vi "Modify Custom Waveform.vi"(11 "Custom Wfm Config":T1={"File Path"="", "Sample Rate (Hz)"=10000000.0, "Read From"=0, "Pre Delay (s)"=0.0, "Post Delay (s)"=0.0, "Scale"=1.0} {"Scale" min=0.0 format="%#_6p"}) -> (2 "Waveform Modified?":bool, 3 "Modified Waveform":waveform(dbl))   [LabVIEW 2025, in "TDMS Waveform Creator UI.lvlib"]
uses:
  TDMS Waveform Creator UI.lvlib
panel:
  out "File Path":path
  in  "Scale":dbl=1.0 min=0.0 format="%#_6p"
  in  "Post Delay (s)":dbl min=0.0 format="%#_6p"
  in  "Pre Delay (s)":dbl min=0.0 format="%#_6p"
  in  "File Type":enum32{"CSV", "TDMS", "TDM"}(radio)
  in  "Read From":i32 caption="Read From Row/Wfm Index" min=0
  in  "Load File":bool
  in  "Suggest Naming?":bool=TRUE
  in  "Waveform Name":string
  in  "Cancel":bool
  in  "OK":bool
  out "Actual Sample Size":i32
  out "Actual Duration (s)":dbl format="%#_6p"
  out "Waveform Preview":waveform(dbl)(graph)
  in  "Sample Rate (Hz)":dbl=10000000.0 min=0.0 format="%#_6p"
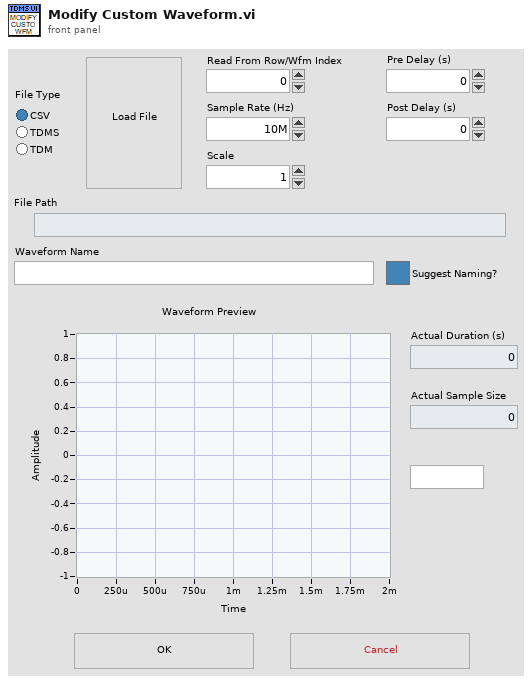
[diagram p1: front panel]
types:
  T1 = cluster{"File Path":string, "Sample Rate (Hz)":dbl, "Read From":i32, "Pre Delay (s)":dbl, "Post Delay (s)":dbl, "Scale":dbl}
  T2 = cluster{"pattern (all files)":string, "pattern label":string, "prompt":string}
  T3 = cluster{"pattern (all files)":string, "pattern label":string, "prompt":string}[]
  T4 = enum8{"Enabled", "Disabled", "Disabled and Grayed Out"}
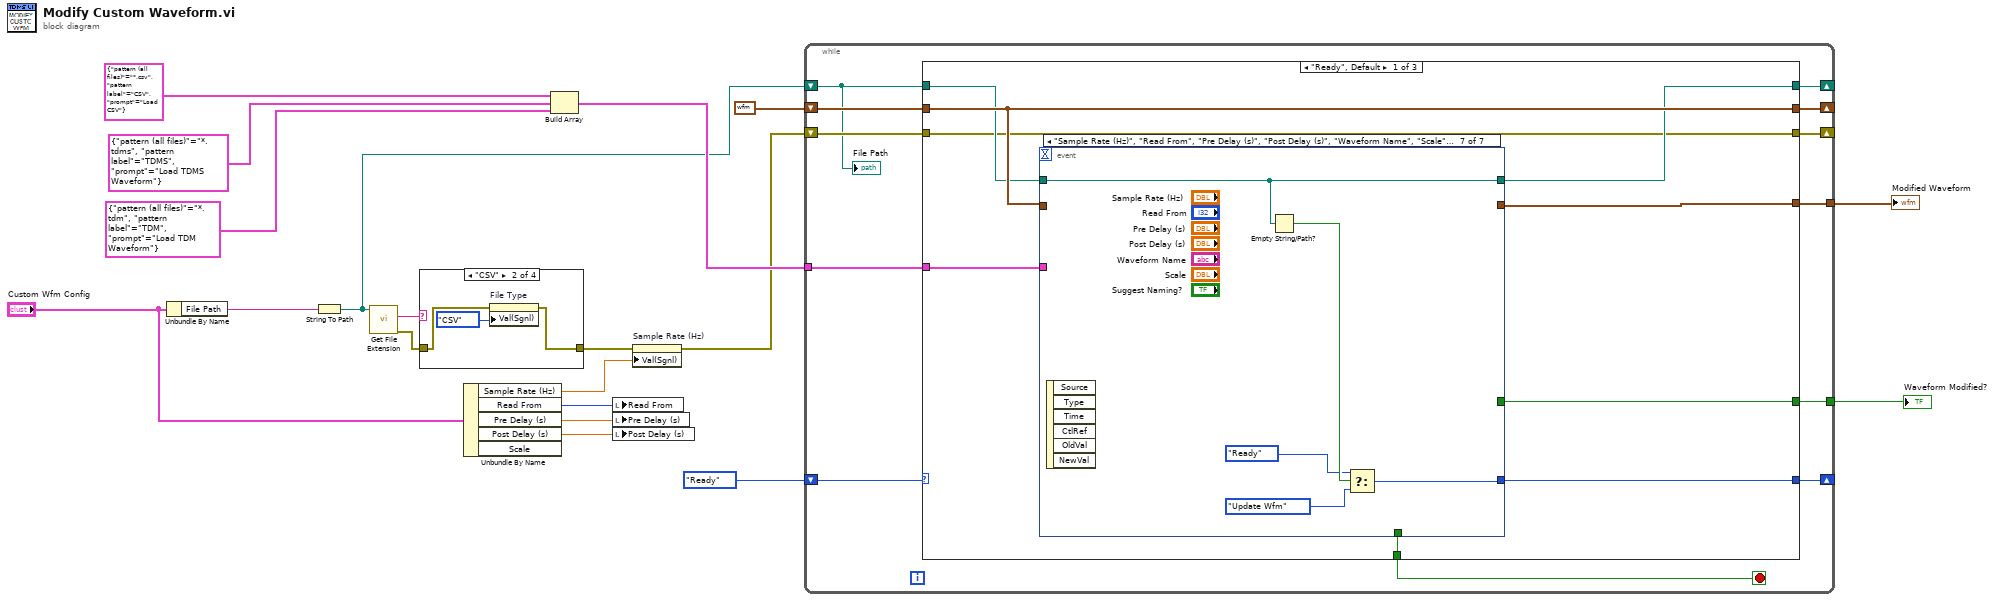
[diagram p0: block diagram]
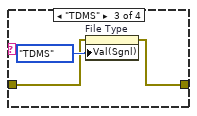
[diagram p3: hidden frame]
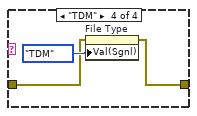
[diagram p4: hidden frame]
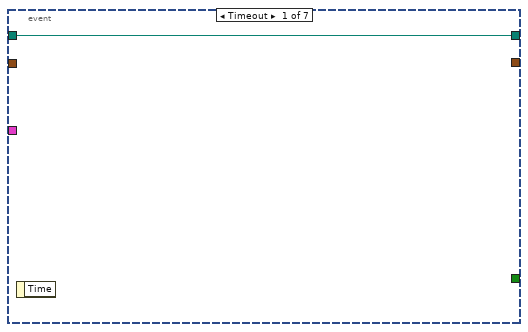
[diagram p5: hidden frame]
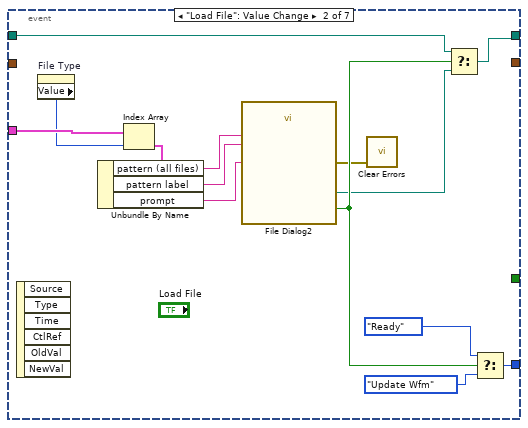
[diagram p6: hidden frame]
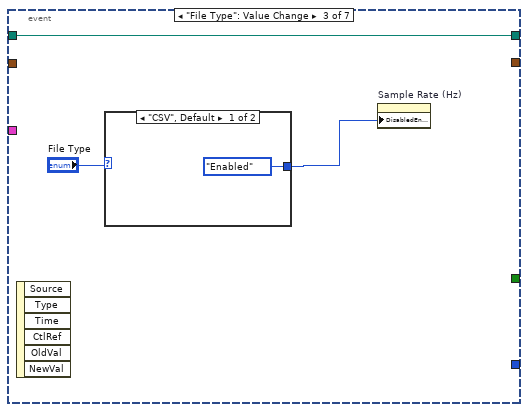
[diagram p7: hidden frame]
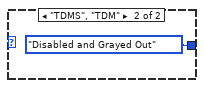
[diagram p8: hidden frame]
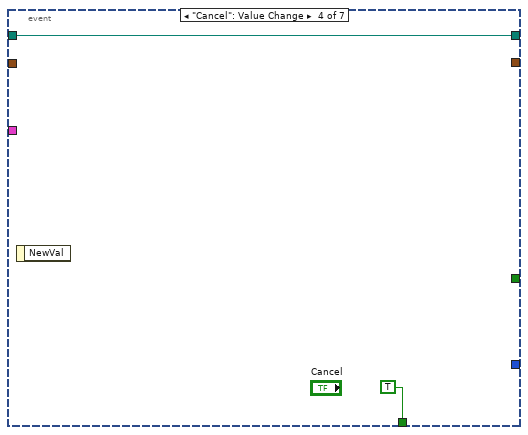
[diagram p9: hidden frame]
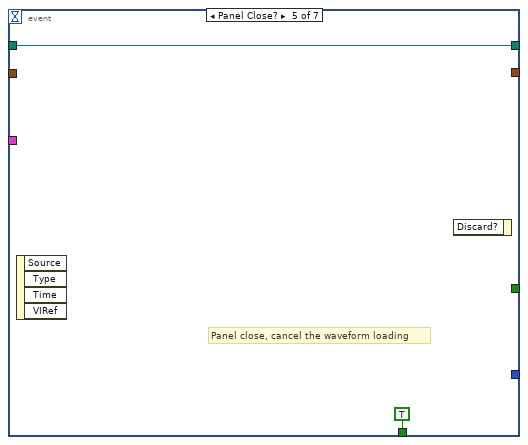
[diagram p10: hidden frame]
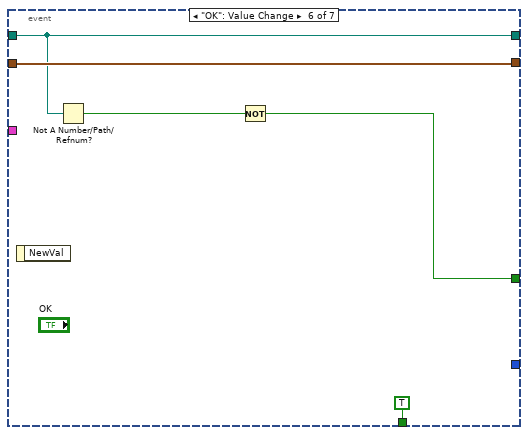
[diagram p11: hidden frame]
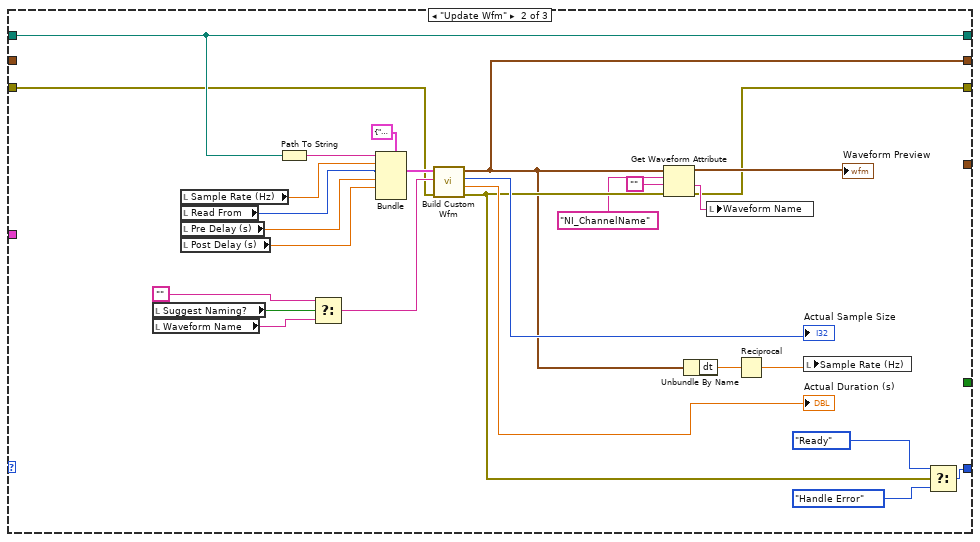
[diagram p12: hidden frame]
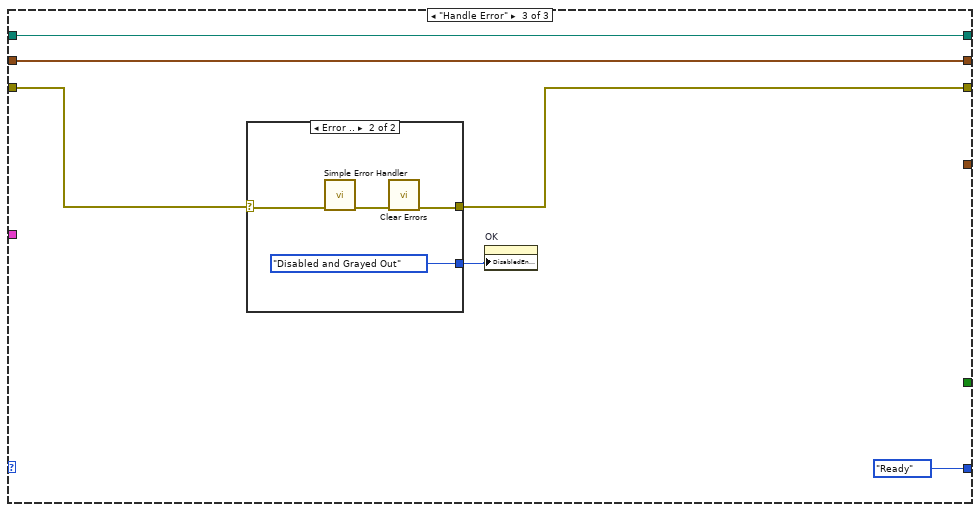
[diagram p13: hidden frame]
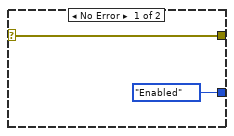
[diagram p14: hidden frame]
diagram:
  n1 = Unbundle By Name("Custom Wfm Config") -> ("File Path"=w11:string)
  n2 = String To Path(string=w11) -> (path=w10:path)
  n3 = call <vilib>:"Get File Extension.vi"("file"=w10) -> ("error out"=w8:errorcluster, "lowercase file extension"=w9:string)  [unwired: 6 in, 3 out]
  n4 = case shown="\"CSV\"" w9 {
    tunnel: w8 -> [w20 w21 w24 w27]
    tunnel: [w20 w22 w25 w28] -> w7
    frame Default {
    }
    frame "CSV" {
      n5 = property on="File Type" class="RadioBtnsControl (strict)"(error in=w21, "Val(Sgnl)"=enum32{"CSV", "TDMS", "TDM"}."CSV" ("Value (Signaling)")) -> (error out=w22:errorcluster)  [unwired: 1 in, 1 out]
    }
    frame "TDMS" {
      n6 = property on="File Type" class="RadioBtnsControl (strict)"(error in=w24, "Val(Sgnl)"=enum32{"CSV", "TDMS", "TDM"}."TDMS" ("Value (Signaling)")) -> (error out=w25:errorcluster)  [unwired: 1 in, 1 out]
    }
    frame "TDM" {
      n7 = property on="File Type" class="RadioBtnsControl (strict)"(error in=w27, "Val(Sgnl)"=enum32{"CSV", "TDMS", "TDM"}."TDM" ("Value (Signaling)")) -> (error out=w28:errorcluster)  [unwired: 1 in, 1 out]
    }
  }
  n8 = Unbundle By Name("Custom Wfm Config") -> ("Sample Rate (Hz)"=w4:dbl, "Read From"=w3:i32, "Pre Delay (s)"=w2:dbl, "Post Delay (s)"=w1:dbl)  [unwired: 1 out]
  n9 = Build Array(T2 {"pattern (all files)"="*.csv", "pattern label"="CSV", "prompt"="Load CSV"}, T2 {"pattern (all files)"="*.tdms", "pattern label"="TDMS", "prompt"="Load TDMS Waveform"}, T2 {"pattern (all files)"="*.tdm", "pattern label"="TDM", "prompt"="Load TDM Waveform"}) -> (w13:T3)
  n10 = local write "Read From"(w3) -> ()
  n11 = local write "Pre Delay (s)"(w2) -> ()
  n12 = local write "Post Delay (s)"(w1) -> ()
  n13 = property on="Sample Rate (Hz)" class="DigNum (strict)"(error in=w7, "Val(Sgnl)"=w4) -> (error out=w6:errorcluster)  [unwired: 1 in, 1 out]
  n14 = while {
    tunnel: [w40] -> w19
    shift-right: [w38] -> _
    shift-left: enum16{"Ready", "Update Wfm", "Handle Error"}."Ready" -> [w39]
    shift-right: [w37] -> _
    shift-left: w10 -> [w30]
    shift-right: [w35] -> _
    shift-left: waveform(dbl) {"t0"=timestamp(0 s since 1904-01-01), "dt"=1.0, "Y"=[]} ("Output Waveform") -> [w36]
    tunnel: [w34] -> w16
    tunnel: w13 -> [w33]
    shift-right: [w31] -> _
    shift-left: w6 -> [w32]
    stop <- w41 stop-if-true
    n15 = case shown="\"Ready\", Default" w39 {
      tunnel: [w50 _ _] -> w41
      tunnel: [w49 _ _] -> w40
      tunnel: [w48 w111 enum16{"Ready", "Update Wfm", "Handle Error"}."Ready"] -> w38
      tunnel: w30 -> [w45 w108 w116]
      tunnel: [w44 w108 w116] -> w37
      tunnel: w36 -> [w47 _ w117]
      tunnel: [w47 w88 w117] -> w35
      tunnel: [w46 _ _] -> w34
      tunnel: w33 -> [w43 _ _]
      tunnel: w32 -> [w42 w91 w114]
      tunnel: [w42 w92 w113] -> w31
      frame "Ready", Default {
        n16 = event shown="[6] \"Sample Rate (Hz)\", \"Read From\", \"Pre Delay (s)\", \"Post Delay (s)\", \"Waveform Name\", \"Scale\", \"Suggest Naming?\": Value Change" {
          selector: _ -> [_ _ _ _ _ _ _]
          dyn-events: _ -> [_ _ _ _ _ _ _]
          timeout: _ -> [_ _ _ _ _ _ _]
          tunnel: [_ _ _ TRUE TRUE TRUE _] -> w50
          tunnel: [_ _ _ _ _ w75 _] -> w49
          tunnel: [_ w65 _ _ _ _ w84] -> w48
          tunnel: w47 -> [_ _ _ _ _ w78 _]
          tunnel: [_ _ _ _ _ w78 _] -> w46
          tunnel: w45 -> [w51 w63 w68 w71 w74 w77 w83]
          tunnel: [w51 w61 w68 w71 w74 w77 w83] -> w44
          tunnel: w43 -> [_ w60 _ _ _ _ _]
          event Timeout {
            n17 = event-data() -> ()  [unwired: 1 in, 1 out]
          }
          event "Load File": Value Change {
            n18 = event-data() -> ()  [unwired: 1 in, 6 out]
            n19 = property on="File Type" class="RadioBtnsControl (strict)"() -> ("Value"=w55:enum32{"CSV", "TDMS", "TDM"})  [unwired: 2 in, 2 out]
            n20 = Index Array(array=w60, index=w55) -> (element=w59:T2)
            n21 = Unbundle By Name(w59) -> ("pattern (all files)"=w58:string, "pattern label"=w57:string, "prompt"=w56:string)
            n22 = call "File Dialog2"("prompt"=w56, "pattern (all files)"=w58, "pattern label"=w57) -> ("selected path"=w62:path, "cancelled"=w64:bool, "error out"=w54:errorcluster)  [unwired: 9 in, 1 out]
            n23 = call <vilib>:"Clear Errors.vi"("error in (no error)"=w54) -> ()  [unwired: 5 in, 2 out]
            n24 = Select(t=w63, s=w64, f=w62) -> (s? t:f=w61:path)
            n25 = Select(t=enum16{"Ready", "Update Wfm", "Handle Error"}."Ready", s=w64, f=enum16{"Ready", "Update Wfm", "Handle Error"}."Update Wfm") -> (s? t:f=w65:enum16{"Ready", "Update Wfm", "Handle Error"})
          }
          event "File Type": Value Change {
            n26 = event-data() -> ()  [unwired: 1 in, 6 out]
            n27 = case shown="\"CSV\", Default" "File Type" {
              tunnel: [T4."Enabled" ("Disabled") T4."Disabled and Grayed Out" ("Disabled")] -> w67
              frame "CSV", Default {
              }
              frame "TDMS", "TDM" {
              }
            }
            n28 = property on="Sample Rate (Hz)" class="DigNum (strict)"("DisabledEnum"=w67) -> ()  [unwired: 2 in, 2 out]
          }
          event "Cancel": Value Change {
            n29 = event-data() -> ()  [unwired: 1 in, 1 out]
          }
          event Panel Close? {
            # "Panel close, cancel the waveform loading"
            n30 = event-data() -> ()  [unwired: 1 in, 4 out]
            n31 = event-data() -> ()  [unwired: 2 in, 1 out]
          }
          event "OK": Value Change {
            n32 = event-data() -> ()  [unwired: 1 in, 1 out]
            n33 = Not A Number/Path/Refnum?(number/path/refnum=w77) -> (NaN/Path/Refnum?=w76:bool)
            n34 = Not(x=w76) -> (.not. x?=w75:bool)
          }
          event "Sample Rate (Hz)", "Read From", "Pre Delay (s)", "Post Delay (s)", "Waveform Name", "Scale", "Suggest Naming?": Value Change {
            n35 = event-data() -> ()  [unwired: 1 in, 6 out]
            n36 = Empty String/Path?(string/path=w83) -> (empty?=w82:bool)
            n37 = Select(t=enum16{"Ready", "Update Wfm", "Handle Error"}."Ready", s=w82, f=enum16{"Ready", "Update Wfm", "Handle Error"}."Update Wfm") -> (s? t:f=w84:enum16{"Ready", "Update Wfm", "Handle Error"})
          }
        }
      }
      frame "Update Wfm" {
        n38 = local read "Suggest Naming?"() -> (w97:bool)
        n39 = local read "Waveform Name"() -> (w93:string)
        n40 = local read "Sample Rate (Hz)"() -> (w107:dbl)
        n41 = local read "Read From"() -> (w106:i32)
        n42 = local read "Pre Delay (s)"() -> (w105:dbl)
        n43 = local read "Post Delay (s)"() -> (w104:dbl)
        n44 = Path To String(path=w108) -> (string=w85:string)
        n45 = Select(t="", s=w97, f=w93) -> (s? t:f=w103:string)
        n46 = Bundle(cluster=T1 {"File Path"="", "Sample Rate (Hz)"=10000000.0, "Read From"=0, "Pre Delay (s)"=0.0, "Post Delay (s)"=0.0, "Scale"=1.0} ("Custom Wfm Config"), "File Path"=w85, "Sample Rate (Hz)"=w107, "Read From"=w106, "Pre Delay (s)"=w105, "Post Delay (s)"=w104) -> (w109:T1)  [unwired: 1 in]
        n47 = call "Build Custom Wfm.vi"("error in"=w91, "User Provided Name"=w103, "Custom Wfm Config"=w109) -> ("error out"=w99:errorcluster, "Actual Duration (s)"=→"Actual Duration (s)":dbl, "Actual Sample Size"=→"Actual Sample Size":i32, "Waveform"=w88:waveform(dbl))  [unwired: 5 in]
        n48 = Get Waveform Attribute(4:w99, 5:"", 6:"NI_ChannelName" ("name"), 7:w88) -> (0:w92:errorcluster, 1:w94:string, 3:→"Waveform Preview":waveform(dbl))  [unwired: 1 out]
        n49 = Unbundle By Name(w88) -> ("dt"=w87:dbl)
        n50 = local write "Waveform Name"(w94) -> ()
        n51 = Reciprocal(x=w87) -> (1/x=w86:dbl)
        n52 = local write "Sample Rate (Hz)"(w86) -> ()
        n53 = Select(t=enum16{"Ready", "Update Wfm", "Handle Error"}."Ready", s=w99, f=enum16{"Ready", "Update Wfm", "Handle Error"}."Handle Error") -> (s? t:f=w111:enum16{"Ready", "Update Wfm", "Handle Error"})
      }
      frame "Handle Error" {
        n54 = case shown="Error .." w114 {
          selector: w114 -> [w119 w123]
          tunnel: [w119 w120] -> w113
          tunnel: [T4."Enabled" ("DisabledEnum") T4."Disabled and Grayed Out" ("DisabledEnum")] -> w115
          frame No Error {
          }
          frame Error {
            n55 = call <vilib>:"Simple Error Handler.vi"("error in (no error)"=w123) -> ("error out"=w122:errorcluster)  [unwired: 4 in, 4 out]
            n56 = call <vilib>:"Clear Errors.vi"("error in (no error)"=w122) -> ("error out"=w120:errorcluster)  [unwired: 5 in, 1 out]
          }
        }
        n57 = property on="OK" class="Bool"("DisabledEnum"=w115) -> ()  [unwired: 2 in, 2 out]
      }
    }
    "File Path" <- w30
  }
  "Waveform Modified?" <- w19
  "Modified Waveform" <- w16
